vi "String info.vi"(8 "error in (no error)":errorcluster, 11 "Variant":variant) -> (0 "error out":errorcluster, 3 "child strings":string[](array[string]))   [LabVIEW 2017, in "DSF Configuration Utility.lvlib"]
uses:
  DSF Configuration.llb/DSF Configuration Utility.lvlib
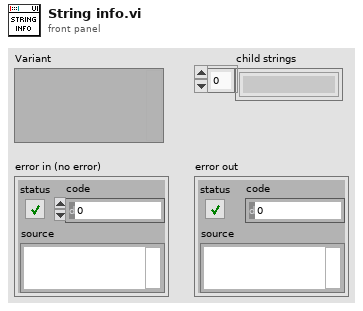
[diagram p1: front panel]
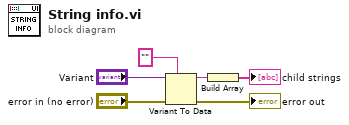
[diagram p0: block diagram]
diagram:
  n1 = Variant To Data(error in="error in (no error)", type="", Variant="Variant") -> (data=w3:string, error out=→"error out":errorcluster)
  n2 = Build Array(w3) -> (→"child strings":string[])
